vi "Do.vi"(8 "error in (no error)":errorcluster, 10 "Actor in":refnum<class "Actor.lvclass">, 11 "Nested Value Update Msg":refnum<class "Nested Value Update Msg.lvclass">) -> (0 "error out":errorcluster, 2 "Actor out":refnum<class "Actor.lvclass">)   [LabVIEW 2020, in "MVA Framework.lvlib" / "IViewable.lvlib" / "Nested Value Update Msg.lvclass"]
doc: "This VI delivers the message to the actor by calling the appropriate method(s) on the actor."
uses:
  Nested Value Update Msg.lvclass
  <vilib>/ActorFramework/Actor/Actor.lvclass
  IViewable/IViewable.lvclass
  C:/Program Files/National Instruments/LabVIEW 2020/vi.lib/ActorFramework/Actor/Actor.lvclass
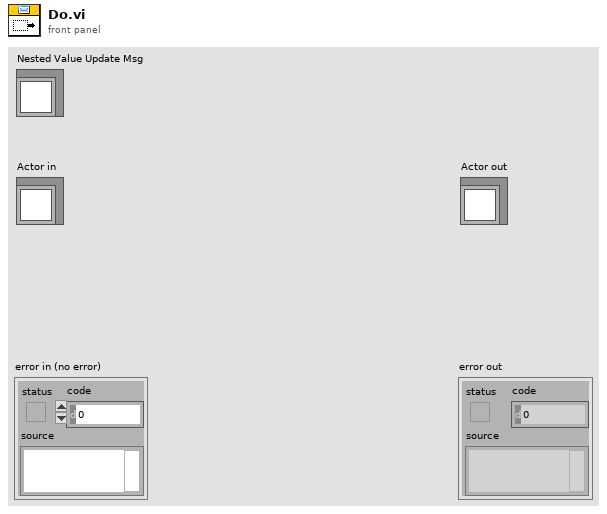
[diagram p1: front panel]
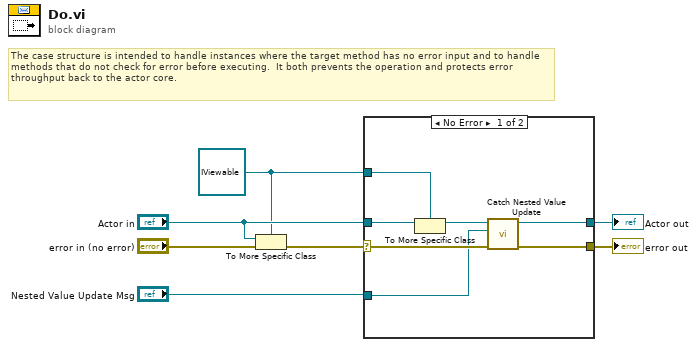
[diagram p0: block diagram]
diagram:
  w1 = refnum<class "IViewable.lvclass"> refnum ("Actor in")
  # "The case structure is intended to handle instances where the target method has no error input and to handle methods that do not check for error before executing.  It both prevents the operation and protects error throughput back to the actor core."
  n1 = To More Specific Class(target class=w1, reference="Actor in", error in="error in (no error)") -> (error out=w5:errorcluster)  [unwired: 1 out]
  n2 = case shown="No Error" w5 {
    selector: w5 -> [w12 w16]
    tunnel: [w14 w16] -> w4
    tunnel: [w13 w15] -> w3
    tunnel: "Actor in" -> [w11 w15]
    tunnel: w1 -> [w10 _]
    tunnel: "Nested Value Update Msg" -> [w8 _]
    frame No Error {
      n3 = To More Specific Class(target class=w10, reference=w11) -> (specific class reference=w9:refnum<class "IViewable.lvclass">)  [unwired: 1 in, 1 out]
      n4 = call-dynamic "Catch Nested Value Update.vi"("error in (no error)"=w12, "Nested Value Update Msg"=w8, "IViewable In"=w9) -> ("error out"=w14:errorcluster, "IViewable Out"=w13:refnum<class "IViewable.lvclass">)  [unwired: 7 in]
    }
    frame Error {
      # "If type check fails, pass the\noriginal object out again."
    }
  }
  "error out" <- w4
  "Actor out" <- w3
